vi "CommitParameters.vi"(8 "error in":errorcluster, 11 "camera handle in":i64) -> (0 "error out":errorcluster, 3 "camera handle out":i64)   [LabVIEW 2019, in "PICam.lvlib"]
uses:
  PICam.lvlib
  Picam64.dll
panel:
  out "piint* (failed_parameter_count)":i64
  out "PicamParameter** (failed_parameter_array)":u64
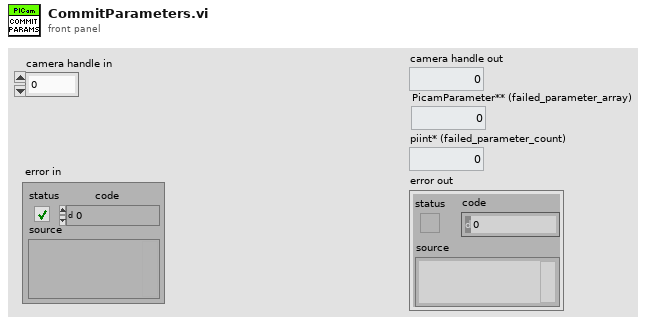
[diagram p1: front panel]
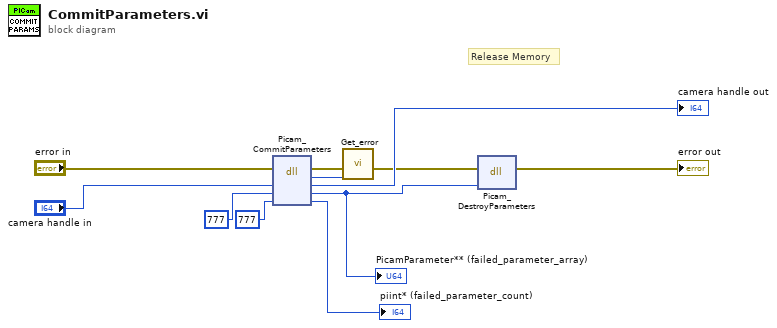
[diagram p0: block diagram]
diagram:
  # "Release Memory"
  n1 = dll-call lib="Picam*.*" fn="Picam_CommitParameters"(error in="error in", "PicamHandle (camera_or_accessory)"="camera handle in", "PicamParameter** (failed_parameter_array)"=u64 777, "piint* (failed_parameter_count)"=i64 777) -> (error out=w8:errorcluster, "error"=w7:u64, "PicamHandle (camera_or_accessory)"=→"camera handle out":i64, "PicamParameter** (failed_parameter_array)"=w2:u64, "piint* (failed_parameter_count)"=→"piint* (failed_parameter_count)":u64)  [unwired: 2 in, 1 out]
  "PicamParameter** (failed_parameter_array)" <- w2
  n2 = call "Get_error.vi"("PICam_Error"=w7, "error in (no error)"=w8) -> ("error out"=w4:errorcluster)  [unwired: 9 in]
  n3 = dll-call lib="Picam*.*" fn="Picam_DestroyParameters"(error in=w4, "PicamParameter* (parameters)"=w2) -> (error out=→"error out":errorcluster)  [unwired: 4 in, 1 out]
